vi "PDFContentByte Fill Color.vi"(0 "PDFContentByte":refnum<k24>, 2 "CB SetColor":T1, 11 "error in (no error)":errorcluster, 13 "Color Box":u32(colorbox)=16777222) -> (4 "PDFContentByte duplicate":refnum<k24>, 15 "error out":errorcluster)   [LabVIEW 2013]
doc: "Version 1.0\nDeveloped by Jean-Marc Simard\nCopyright © 2010, Exaprom Inc.\nAll rights reserved.\nLicense: BSD\n\nWith iTextSharp 4.1.6 (http://itextsharp.sourceforge.net)\nunder Mozilla Public License Version 1.1\n(http://www.mozilla.org/MPL/MPL-1.1.html)"
uses:
  C:/Users/MaxCorp/Documents/GitHub/TopView/DLL/itextsharp.dll
  DLL/itextsharp.dll
  Controls/CB SetColor.ctl
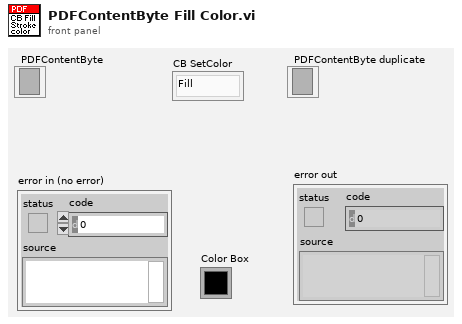
[diagram p1: front panel]
types:
  T1 = typedef "CB SetColor.ctl" = enum16{"Fill", "Stroke"}
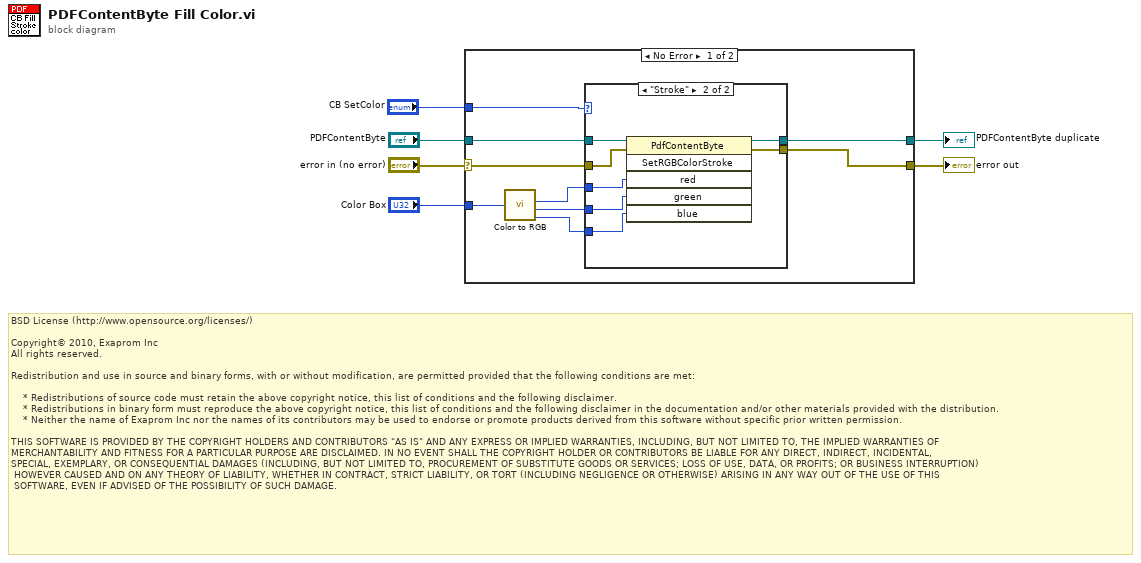
[diagram p0: block diagram]
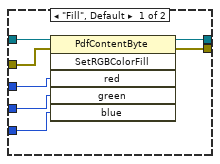
[diagram p2: hidden frame]
diagram:
  # "BSD License (http://www.opensource.org/licenses/)\n\nCopyright© 2010, Exaprom Inc\nAll rights reserved.\n\nRedistribution and use in source and binary forms, with or without modification, are permitted provided that the following conditions are met:\n\n    * Redistributions of source code must retain the above copyright notice, this list of conditions and the following disclaimer.\n    * Redistributions in binary form must reproduce the above copyright notice, this list of conditions and the following disclaimer in the documentation and/or other materials provided with the distribution.\n    * Neither the name of Exaprom Inc nor the names of its contributors may be used to endorse or promote products derived from this software without specific prior written permission.\n\nTHIS SOFTWARE IS PROVIDED BY THE COPYRIGHT HOLDERS AND CONTRIBUTORS \"AS IS\" AND ANY EXPRESS OR IMPLIED WARRANTIES, INCLUDING, BUT NOT LIMITED TO, THE IMPLIED WARRANTIES OF \nMERCHANTABILITY AND FITNESS FOR A PARTICULAR PURPOSE ARE DISCLAIMED. IN NO EVENT SHALL THE COPYRIGHT HOLDER OR CONTRIBUTORS BE LIABLE FOR ANY DIRECT, INDIRECT, INCIDENTAL,\nSPECIAL, EXEMPLARY, OR CONSEQUENTIAL DAMAGES (INCLUDING, BUT NOT LIMITED TO, PROCUREMENT OF SUBSTITUTE GOODS OR SERVICES; LOSS OF USE, DATA, OR PROFITS; OR BUSINESS INTERRUPTION)\n HOWEVER CAUSED AND ON ANY THEORY OF LIABILITY, WHETHER IN CONTRACT, STRICT LIABILITY, OR TORT (INCLUDING NEGLIGENCE OR OTHERWISE) ARISING IN ANY WAY OUT OF THE USE OF THIS\n SOFTWARE, EVEN IF ADVISED OF THE POSSIBILITY OF SUCH DAMAGE."
  n1 = case shown="No Error" "error in (no error)" {
    selector: "error in (no error)" -> [w7 w30]
    tunnel: "PDFContentByte" -> [w15 w31]
    tunnel: [w14 w31] -> w3
    tunnel: [w12 w30] -> w5
    tunnel: "Color Box" -> [w8 _]
    tunnel: "CB SetColor" -> [w13 _]
    frame No Error {
      n2 = call <vilib>:"Color to RGB.vi"("Color"=w8) -> ("R"=w10:u8, "G"=w11:u8, "B"=w9:u8)  [unwired: 1 out]
      n3 = case shown="\"Stroke\"" w13 {
        tunnel: w15 -> [w22 w29]
        tunnel: [w21 w28] -> w14
        tunnel: [w20 w27] -> w12
        tunnel: w11 -> [w18 w26]
        tunnel: w10 -> [w19 w25]
        tunnel: w9 -> [w17 w24]
        tunnel: w7 -> [w16 w23]
        frame "Fill", Default {
          n4 = invoke class="PdfContentByte" method="SetRGBColorFill"(reference=w22, error in=w16, "red"=w19, "green"=w18, "blue"=w17) -> (reference out=w21:refnum<k24>, error out=w20:errorcluster)  [unwired: 1 in, 4 out]
        }
        frame "Stroke" {
          n5 = invoke class="PdfContentByte" method="SetRGBColorStroke"(reference=w29, error in=w23, "red"=w25, "green"=w26, "blue"=w24) -> (reference out=w28:refnum<k24>, error out=w27:errorcluster)  [unwired: 1 in, 4 out]
        }
      }
    }
    frame Error {
    }
  }
  "PDFContentByte duplicate" <- w3
  "error out" <- w5
